vi "Write I64.vi"(8 "error in (no error)":errorcluster, 9 "Numeric":i64, 10 "Key":string="myhome/kitchen/temp", 11 "Zenoh in":refnum<class "Zenoh.lvclass">) -> (0 "error out":errorcluster)   [LabVIEW 2021, in "Zenoh.lvclass"]
doc: "Flatten an I64 and write to zenoh with provided key."
uses:
  Zenoh.lvclass
  Zenoh.lvclass/Zenoh.ctl
  <vilib>/CIF Foundation/CIF Utilities/DataTypes/Typedef/Endian.ctl
  SubVIs/Get Zenoh Path.vi
  <vilib>/CIF Foundation/CIF Utilities/DataTypes/DataTypes_CIF_U.lvlib
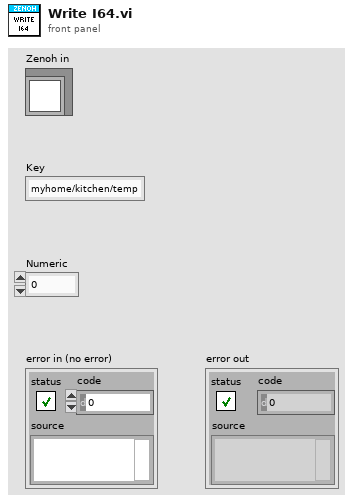
[diagram p1: front panel]
types:
  T1 = typedef "DataTypes_CIF_U.lvlib/Endian.ctl" = enum16{"Little Endian", "Big Endian"}
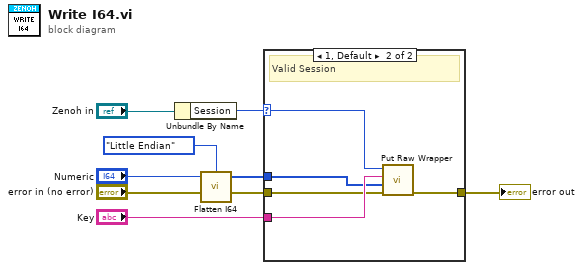
[diagram p0: block diagram]
diagram:
  n1 = Unbundle By Name("Zenoh in") -> ("Session"=w6:u64)
  n2 = call <vilib>:"Flatten I64.vi"("I64"="Numeric", "Endian"=Endian."Little Endian") -> ("Flat Data"=w2:u8[])  [unwired: 3 in]
  n3 = case shown="1, Default" w6 {
    selector: w6 -> [_ w14]
    tunnel: "Key" -> [_ w13]
    tunnel: "error in (no error)" -> [w9 w12]
    tunnel: [w9 w10] -> w5
    tunnel: w2 -> [_ w11]
    frame 0 {
      # "Invalid session"
    }
    frame 1, Default {
      # "Valid Session"
      n4 = call "Put Raw Wrapper.vi"("error in (no error)"=w12, "Raw Data"=w11, "key"=w13, "Session in"=w14) -> ("error out"=w10:errorcluster)  [unwired: 7 in]
    }
  }
  "error out" <- w5
